vi "Events With Slow Digital Input.vi"() -> ()   [LabVIEW 2013]
uses:
  Version Token.ctl
  APU/Settings.ctl
  APU/Input.ctl
  APU/Output.ctl
  APU/Shared Settings.ctl
  ECU Event/Timing/Measure Output.ctl
  ECU Event/Timing/Measure Settings.ctl
  ECU Event/Timing/Capture Output.ctl
  <vilib>/Platform/TimedLoop/XDataNode/timing_clust.ctl
  <vilib>/Platform/TimedLoop/XDataNode/nitl_modes.ctl
  <vilib>/Platform/TimedLoop/XDataNode/wakeup.ctl
  ECU Event/Timing/Capture Settings.ctl
  <vilib>/rvi/Emulation/niFpgaSctlEmulationGetInTimedLoop.vi
  <vilib>/rvi/Emulation/niFpgaEmulationReportErrorSimple.vi
  <vilib>/rvi/Emulation/niFpgaGetClockAttributes.vi
  <vilib>/rvi/Emulation/niFpgaCriticalErrorInLSC.vi
  <vilib>/rvi/eio/common/nirviEmuTemplateMethod_errors.vi
  ECU Event/Timing/Measure Events (Non-40MHz).vi
  <vilib>/Platform/TimedLoop/XDataNode/XDataNode.xnode
  <vilib>/eio/EIONode/EIONode.xnode
  APU/APU.lvlib
  <vilib>/Platform/TimedLoop/XDataNode/XDNodeRunTimeDep.lvlib
  ECU Event/Timing/ECU Event Timing.lvlib
  Engine Simulation Toolkit.lvlib
panel:
  in  "go.apu 1":bool
  out "capture.Multi Event DIO 15.Event 4":T1
  out "capture.Multi Event DIO 15.Event 3":T1
  out "capture.Multi Event DIO 15.Event 2":T1
  out "capture.Multi Event DIO 14.Event 4":T1
  out "capture.Multi Event DIO 14.Event 3":T1
  out "capture.Multi Event DIO 14.Event 2":T1
  out "capture.Multi Event DIO 13.Event 4":T1
  out "capture.Multi Event DIO 13.Event 3":T1
  out "capture.Multi Event DIO 13.Event 2":T1
  out "capture.Multi Event DIO 12.Event 4":T1
  out "capture.Multi Event DIO 12.Event 3":T1
  out "capture.Multi Event DIO 12.Event 2":T1
  out "capture.Multi Event DIO 11.Event 4":T1
  out "capture.Multi Event DIO 11.Event 3":T1
  out "capture.Multi Event DIO 11.Event 2":T1
  out "capture.Multi Event DIO 10.Event 4":T1
  out "capture.Multi Event DIO 10.Event 3":T1
  out "capture.Multi Event DIO 10.Event 2":T1
  out "capture.Multi Event DIO 10.Event 1":T1
  out "capture.Multi Event DIO 11.Event 1":T1
  out "capture.Multi Event DIO 12.Event 1":T1
  out "capture.Multi Event DIO 13.Event 1":T1
  out "capture.Multi Event DIO 14.Event 1":T1
  out "capture.Multi Event DIO 15.Event 1":T1
  in  "settings.Multi Event DIO 10":T2
  in  "settings.Multi Event DIO 11":T2
  in  "settings.Multi Event DIO 12":T2
  in  "settings.Multi Event DIO 13":T2
  in  "settings.Multi Event DIO 14":T2
  in  "settings.Multi Event DIO 15":T2
  out "status.Multi Event DIO 10":T3
  out "status.Multi Event DIO 11":T3
  out "status.Multi Event DIO 12":T3
  out "status.Multi Event DIO 13":T3
  out "status.Multi Event DIO 14":T3
  out "status.Multi Event DIO 15":T3
  out "capture.Event DIO 4.Event 1":T1
  out "capture.Event DIO 5.Event 1":T1
  out "capture.Event DIO 6.Event 1":T1
  out "capture.Event DIO 7.Event 1":T1
  out "capture.Event DIO 8.Event 1":T1
  out "capture.Event DIO 9.Event 1":T1
  in  "settings.Event DIO 4":T2
  in  "settings.Event DIO 5":T2
  in  "settings.Event DIO 6":T2
  in  "settings.Event DIO 7":T2
  in  "settings.Event DIO 8":T2
  in  "settings.Event DIO 9":T2
  out "status.Event DIO 4":T3
  out "status.Event DIO 5":T3
  out "status.Event DIO 6":T3
  out "status.Event DIO 7":T3
  out "status.Event DIO 8":T3
  out "status.Event DIO 9":T3
  in  "shared settings.apu 1":T4 {"cycle start" format="%#.15g"}
  out "output.apu 1":T5 caption="output"
  in  "input.apu 1":T6={"desired speed"=0.0, "reset"=TRUE} caption="input"
  in  "settings.apu 1":T7 caption="settings"
  in  "est.version":T8
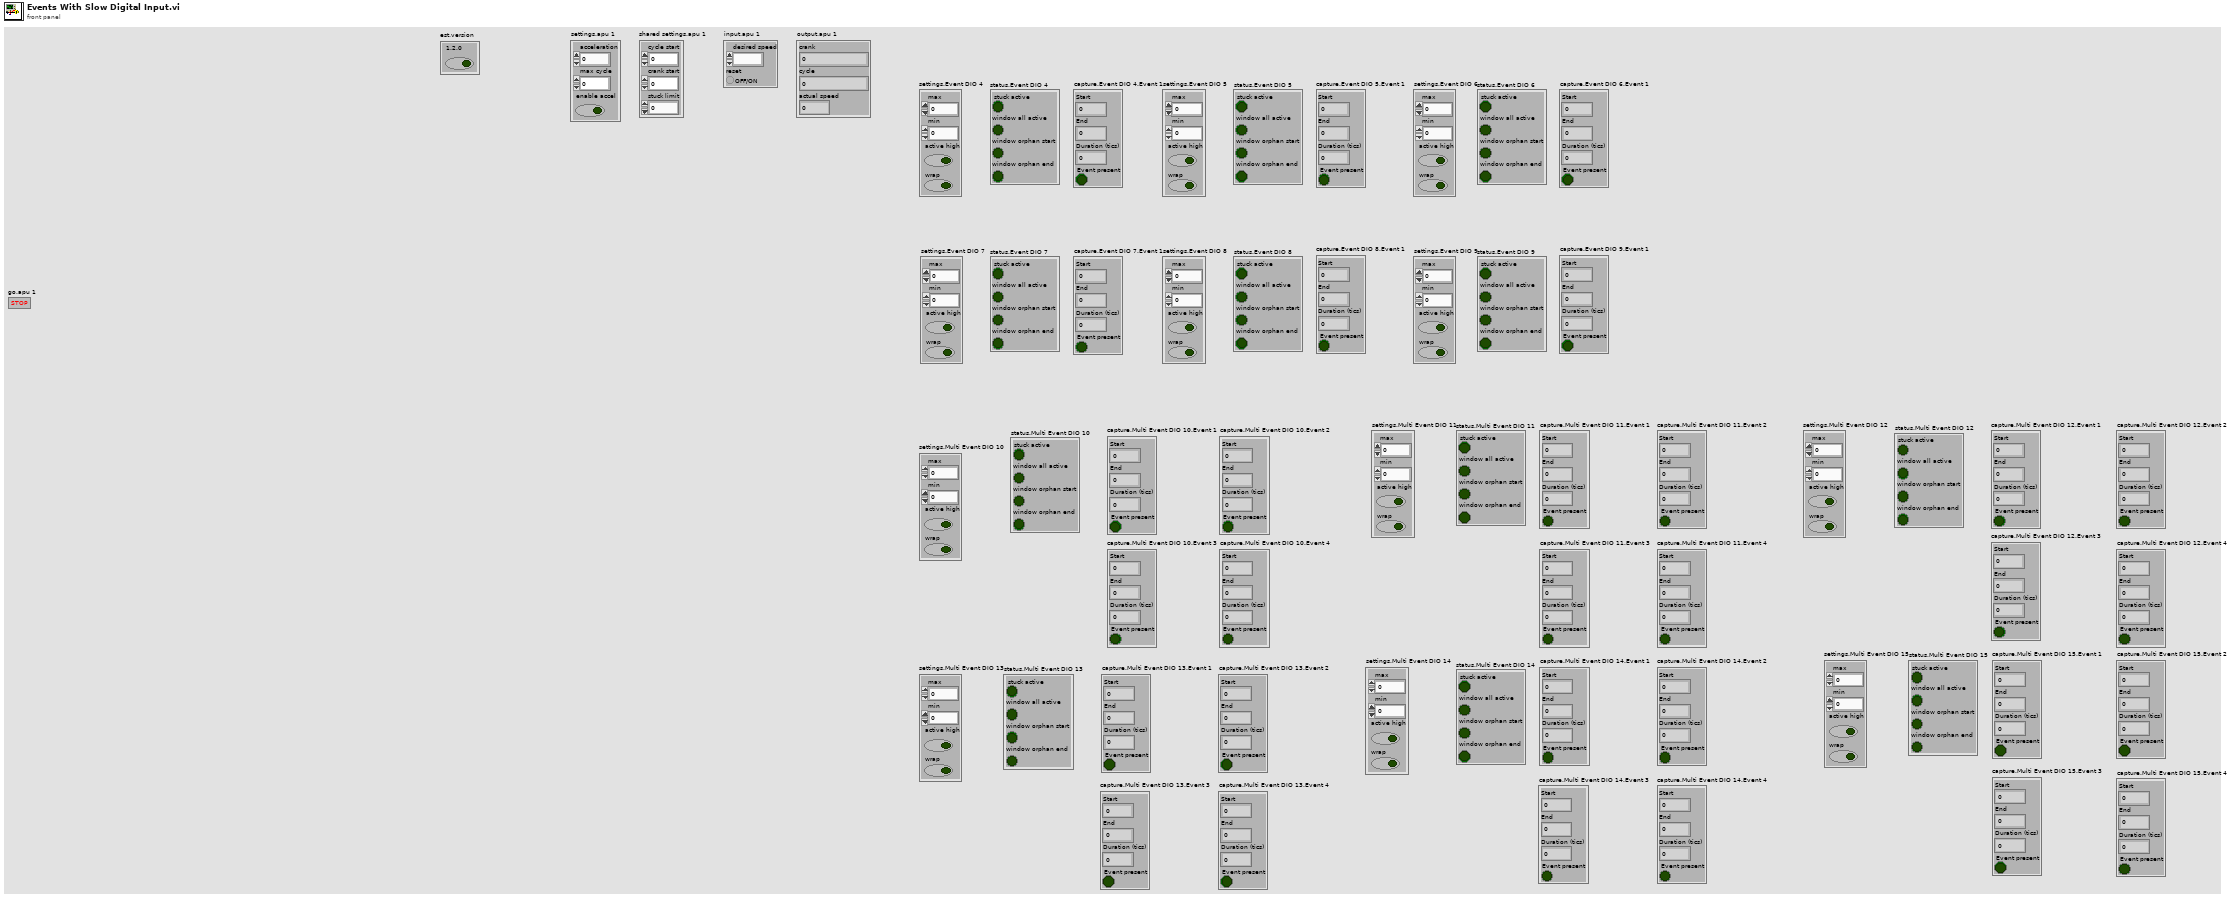
[diagram p1: front panel]
types:
  T1 = typedef "Engine Simulation Toolkit.lvlib/ECU Event Timing.lvlib/Capture Output.ctl" = cluster{"Start":u16, "End":u16, "Duration (tics)":fxp<+,18,18>, "Event present":bool}
  T2 = typedef "Engine Simulation Toolkit.lvlib/ECU Event Timing.lvlib/Measure Settings.ctl" = cluster{"max":u16, "min":u16, "active high":bool, "wrap":bool}
  T3 = typedef "Engine Simulation Toolkit.lvlib/ECU Event Timing.lvlib/Measure Output.ctl" = cluster{"stuck active":bool, "window all active":bool, "window orphan start":bool, "window orphan end":bool}
  T4 = typedef "Engine Simulation Toolkit.lvlib/APU.lvlib/Shared Settings.ctl" = cluster{"cycle start":fxp<+,2,2>, "crank start":u16, "stuck limit":fxp<+,18,18>}
  T5 = typedef "Engine Simulation Toolkit.lvlib/APU.lvlib/Output.ctl" = cluster{"crank":u16, "cycle":u16, "actual speed":fxp<+/-,23,2>}
  T6 = typedef "Engine Simulation Toolkit.lvlib/APU.lvlib/Input.ctl" = cluster{"desired speed":fxp<+/-,23,2>, "reset":bool}
  T7 = typedef "Engine Simulation Toolkit.lvlib/APU.lvlib/Settings.ctl" = cluster{"acceleration":fxp<+,18,-20>, "max cycle":fxp<+,2,2>, "enable accel":bool}
  T8 = typedef "Engine Simulation Toolkit.lvlib/Version Token.ctl" = cluster{"1.2.0":bool}
  T9 = typedef "XDNodeRunTimeDep.lvlib/timing_clust.ctl" = cluster{"Expected End [f-1]":u64, "Actual End [f-1]":u64, "Finished Late? [f-1]":bool, "Expected End [i-1]":u64, "Actual End [i-1]":u64, "Finished Late? [i-1]":bool, "Expected Start [i]":u64, "Actual Start [i]":u64, "Expected Start [f]":u64, "Actual Start [f]":u64, "Source Name":string, "Structure Name":string, "Period":i64, "Deadline":i64, "Offset":i64, "Start":i64, "Priority":i32, "Timeout":i32, "Mode":T10, "Wakeup Reason":T11, "Error":errorcluster, "Source Type":string, "Secondary Source Type":string, "Global End Time":u64, "Global Start Time":u64, "Frame Duration":u64, "Iteration Duration":u64, "Assigned CPU":i32, "I/O Scan Engine Mode":u32}
  T10 = typedef "XDNodeRunTimeDep.lvlib/nitl_modes.ctl" = enum32{"No Change", "Process missed periods, maintain original phase", "Discard missed periods, maintain original phase", "Process missed periods, ignore original phase", "Discard missed periods, ignore original phase"}
  T11 = typedef "XDNodeRunTimeDep.lvlib/wakeup.ctl" = enum32{"Normal", "Aborted", "Asynchronous wakeup", "Timing source error", "Timed loop error", "Timeout"}
  T12 = typedef "Engine Simulation Toolkit.lvlib/APU.lvlib/Register Bus.ctl" = cluster{"Speed":refnum<k21>, "Crank Angle":refnum<k21>, "Cycle Angle":refnum<k21>, "Crank Count":refnum<k21>, "Cycle Count":refnum<k21>, "1.25 MHz Counter":refnum<k21>, "shared settings":T4}
  T13 = typedef "Engine Simulation Toolkit.lvlib/ECU Event Timing.lvlib/Capture Settings.ctl" = u8
  T14 = typedef "Engine Simulation Toolkit.lvlib/ECU Event Timing.lvlib/Measured Data.ctl" = cluster{"start":u16, "end":u16, "duration (tics)":fxp<+,18,18>, "window end":bool, "window begin":bool, "pulse end":bool, "pulse #":u8}
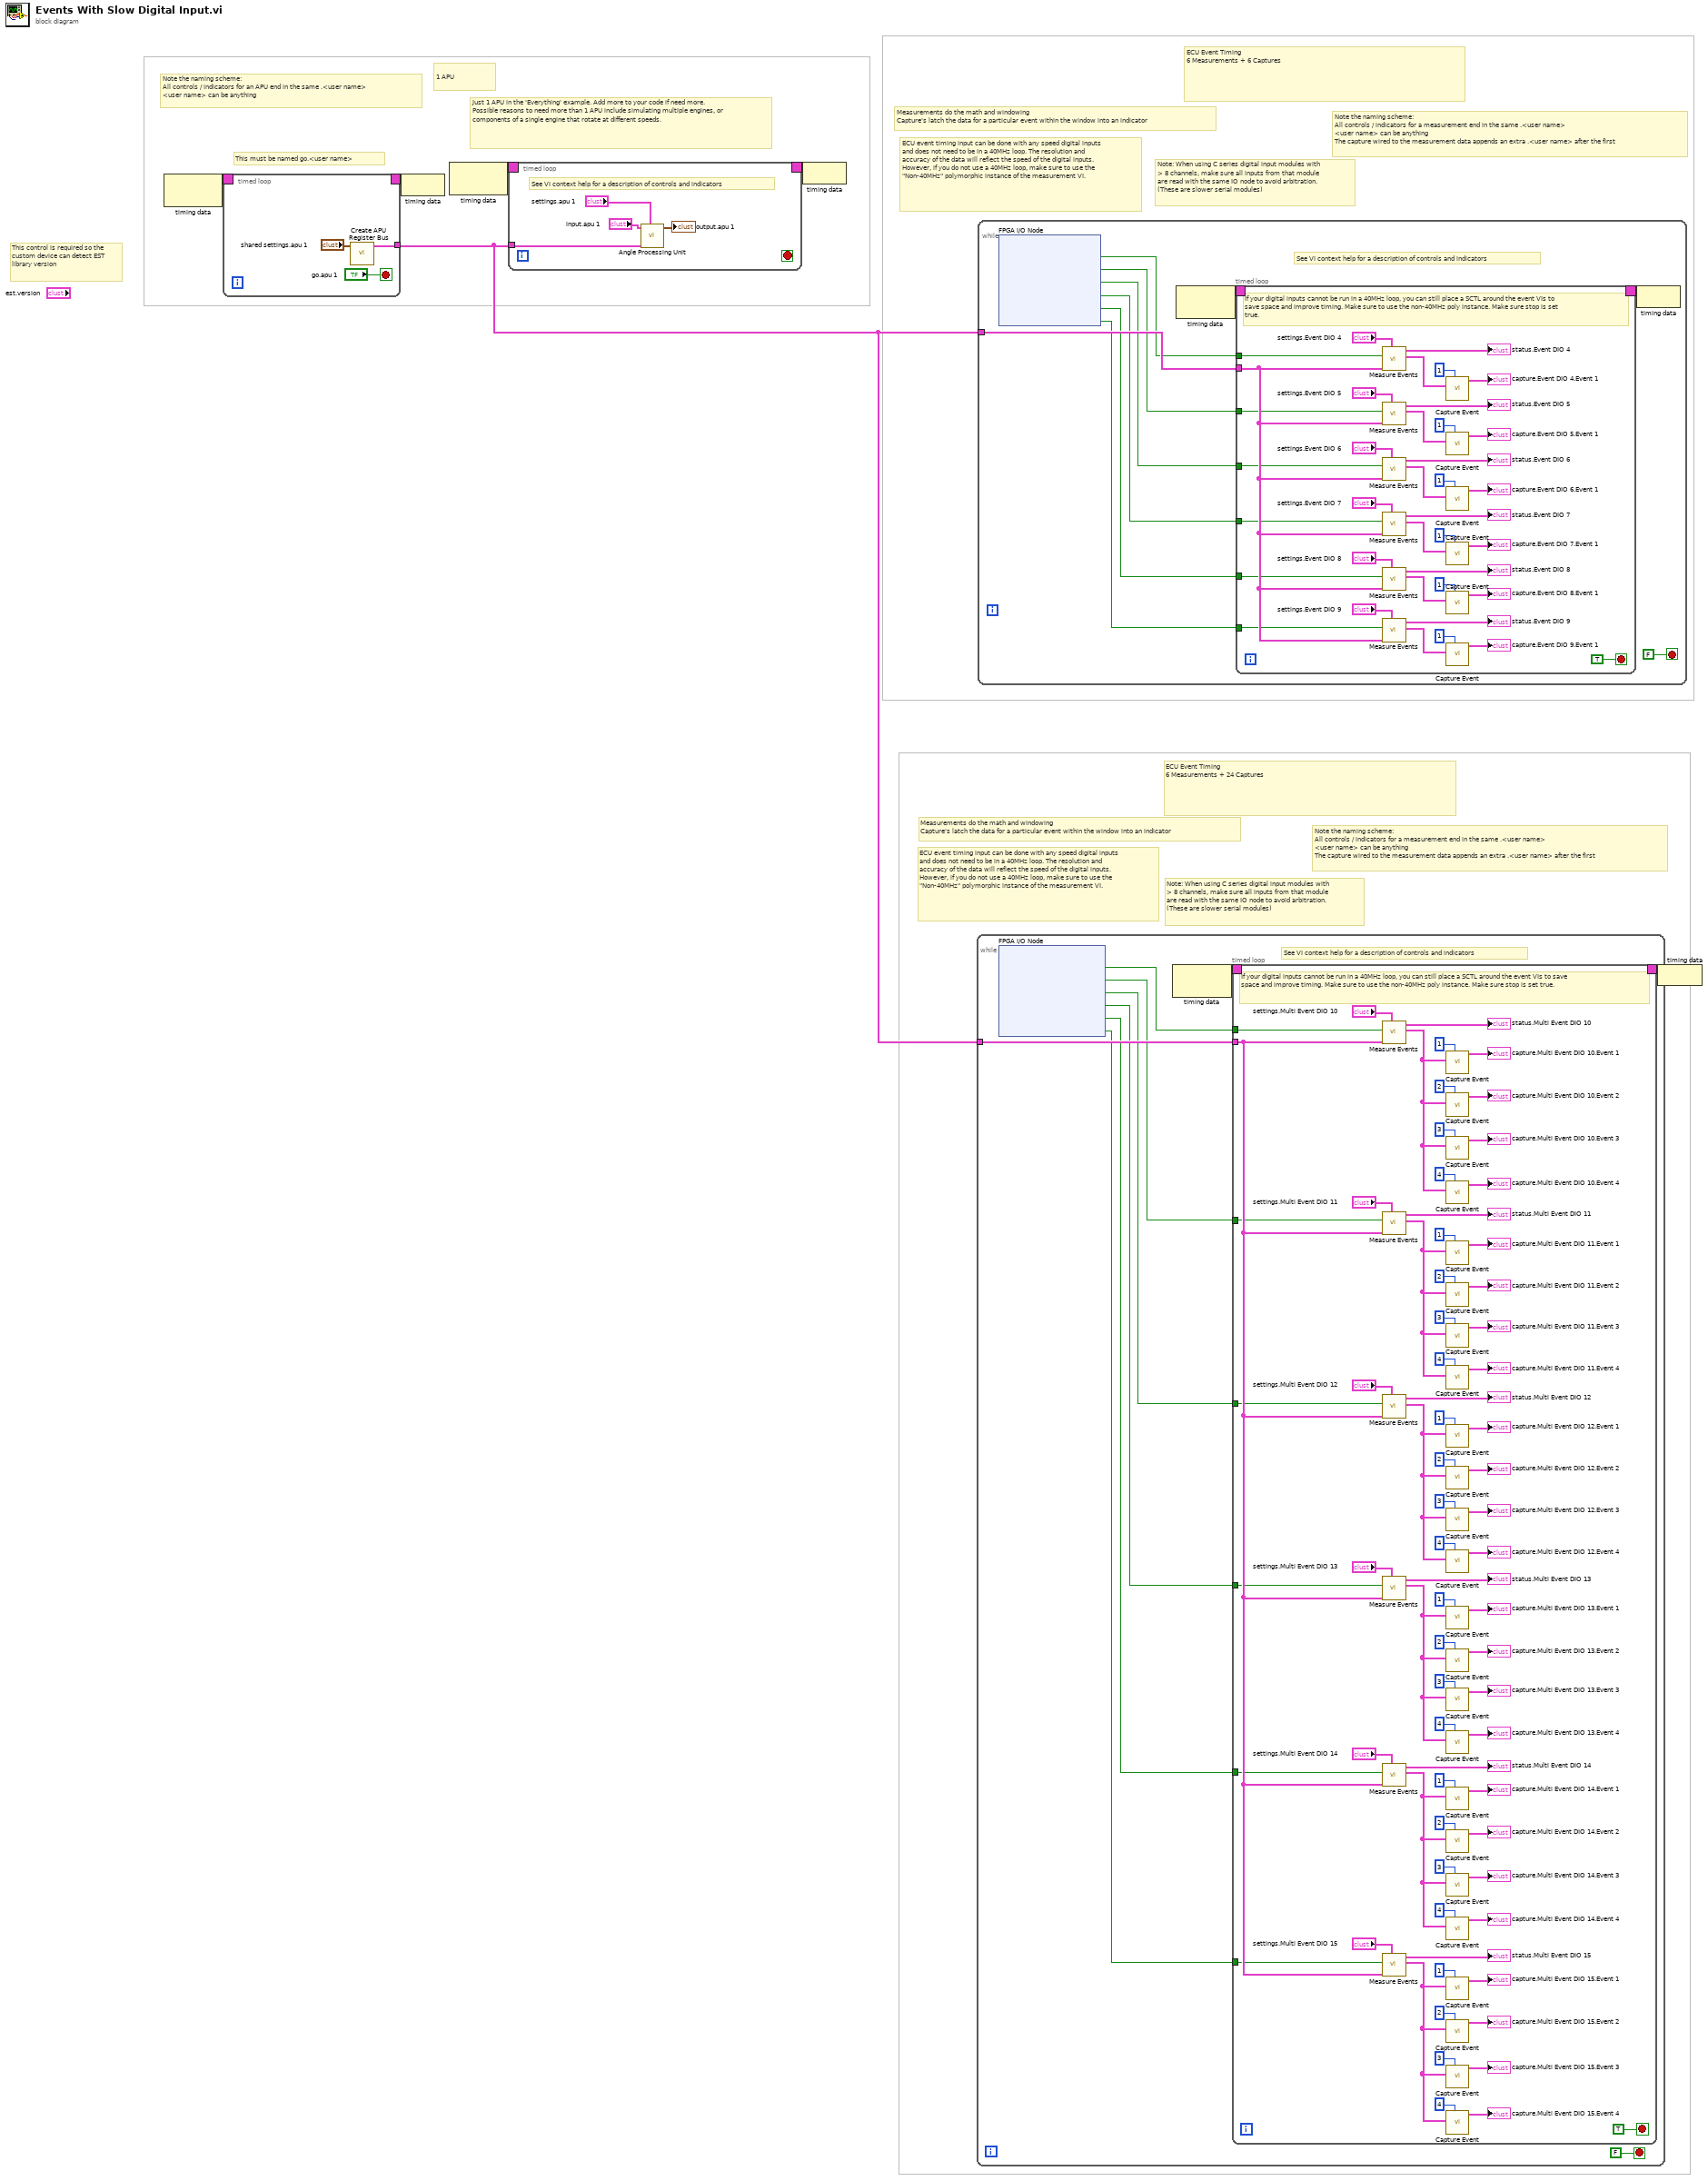
[diagram p0: block diagram]
diagram:
  # "ECU event timing input can be done with any speed digital inputs and does not need to be in a 40MHz loop. The resolution and accuracy of the data will reflect the speed of the digital inputs. However, if you do not use a 40MHz loop, make sure to use the \"Non-40MHz\" polymorphic instance of the measurement VI."
  # "This must be named go.<user name>"
  # "Note: When using C series digital input modules with > 8 channels, make sure all inputs from that module are read with the same IO node to avoid arbitration. (These are slower serial modules)"
  # "Measurements do the math and windowing\nCapture's latch the data for a particular event within the window into an indicator"
  # "ECU Event Timing\n6 Measurements + 24 Captures"
  # "Note the naming scheme: \nAll controls / indicators for a measurement end in the same .<user name>\n<user name> can be anything\nThe capture wired to the measurement data appends an extra .<user name> after the first"
  # "Note: When using C series digital input modules with > 8 channels, make sure all inputs from that module are read with the same IO node to avoid arbitration. (These are slower serial modules)"
  # "Measurements do the math and windowing\nCapture's latch the data for a particular event within the window into an indicator"
  # "ECU Event Timing\n6 Measurements + 6 Captures"
  # "Note the naming scheme: \nAll controls / indicators for a measurement end in the same .<user name>\n<user name> can be anything\nThe capture wired to the measurement data appends an extra .<user name> after the first"
  # "ECU event timing input can be done with any speed digital inputs and does not need to be in a 40MHz loop. The resolution and accuracy of the data will reflect the speed of the digital inputs. However, if you do not use a 40MHz loop, make sure to use the \"Non-40MHz\" polymorphic instance of the measurement VI."
  # "1 APU"
  # "Note the naming scheme: \nAll controls / indicators for an APU end in the same .<user name>\n<user name> can be anything"
  # "Just 1 APU in the 'Everything' example. Add more to your code if need more. Possible reasons to need more than 1 APU include simulating multiple engines, or components of a single engine that rotate at different speeds."
  # "This control is required so the custom device can detect EST library version"
  n1 = node-c288() -> (w2:T9)  [unwired: 1 in]
  n2 = timed-loop {
    timing: w2 -> [_]
    timing-out: [_] -> w1
    tunnel: [w7] -> w3
    stop <- "go.apu 1" stop-if-true
    n3 = call "Create APU Register Bus.vi"("shared settings.<user name>"="shared settings.apu 1") -> ("register bus"=w7:T12)  [unwired: 10 in]
  }
  n4 = node-c288(w1) -> ()
  n5 = node-c288() -> (w5:T9)  [unwired: 1 in]
  n6 = timed-loop {
    timing: w5 -> [_]
    timing-out: [_] -> w4
    tunnel: w3 -> [w11]
    stop <- _ stop-if-true
    # "See VI context help for a description of controls and indicators"
    n7 = call "Angle Processing Unit.vi"("settings.<user name>"="settings.apu 1", "register bus"=w11, "input.<user name>"="input.apu 1") -> ("output.<user name>"=→"output.apu 1":T5)  [unwired: 8 in]
  }
  n8 = node-c288(w4) -> ()
  n9 = while {
    tunnel: w3 -> [w26]
    stop <- FALSE stop-if-true
    # "See VI context help for a description of controls and indicators"
    n10 = xnode "FPGA I/O Node"() -> ("Connector0/DIO10"=w25:bool, "Connector0/DIO11"=w24:bool, "Connector0/DIO12"=w23:bool, "Connector0/DIO13"=w22:bool, "Connector0/DIO14"=w21:bool, "Connector0/DIO15"=w20:bool)  [unwired: 6 in, 6 out]
    n11 = node-c288() -> (w18:T9)  [unwired: 1 in]
    n12 = timed-loop {
      timing: w18 -> [_]
      timing-out: [_] -> w17
      tunnel: w26 -> [w94]
      tunnel: w25 -> [w81]
      tunnel: w24 -> [w80]
      tunnel: w23 -> [w79]
      tunnel: w22 -> [w78]
      tunnel: w21 -> [w77]
      tunnel: w20 -> [w76]
      stop <- TRUE stop-if-true
      # "If your digital inputs cannot be run in a 40MHz loop, you can still place a SCTL around the event VIs to save space and improve timing. Make sure to use the non-40MHz poly instance. Make sure stop is set true."
      n13 = call-poly "Measure Events.vi"("settings.<user name>"="settings.Multi Event DIO 10", "register bus"=w94, "event"=w81) -> ("measured data"=w63:T14, "status.<user name>"=→"status.Multi Event DIO 10":T3)  [unwired: 7 in]
      n14 = call-poly "Measure Events.vi"("settings.<user name>"="settings.Multi Event DIO 11", "register bus"=w94, "event"=w80) -> ("measured data"=w56:T14, "status.<user name>"=→"status.Multi Event DIO 11":T3)  [unwired: 7 in]
      n15 = call-poly "Measure Events.vi"("settings.<user name>"="settings.Multi Event DIO 12", "register bus"=w94, "event"=w79) -> ("measured data"=w49:T14, "status.<user name>"=→"status.Multi Event DIO 12":T3)  [unwired: 7 in]
      n16 = call-poly "Measure Events.vi"("settings.<user name>"="settings.Multi Event DIO 13", "register bus"=w94, "event"=w78) -> ("measured data"=w42:T14, "status.<user name>"=→"status.Multi Event DIO 13":T3)  [unwired: 7 in]
      n17 = call-poly "Measure Events.vi"("settings.<user name>"="settings.Multi Event DIO 14", "register bus"=w94, "event"=w77) -> ("measured data"=w35:T14, "status.<user name>"=→"status.Multi Event DIO 14":T3)  [unwired: 7 in]
      n18 = call-poly "Measure Events.vi"("settings.<user name>"="settings.Multi Event DIO 15", "register bus"=w94, "event"=w76) -> ("measured data"=w28:T14, "status.<user name>"=→"status.Multi Event DIO 15":T3)  [unwired: 7 in]
      n19 = call "Capture Event.vi"("event # to capture"=T13 1 ("Settings.spark 1 shot 1"), "measured data"=w63) -> ("capture.<user name>"=→"capture.Multi Event DIO 10.Event 1":T1)  [unwired: 9 in]
      n20 = call "Capture Event.vi"("event # to capture"=T13 2 ("Settings.spark 1 shot 1"), "measured data"=w63) -> ("capture.<user name>"=→"capture.Multi Event DIO 10.Event 2":T1)  [unwired: 9 in]
      n21 = call "Capture Event.vi"("event # to capture"=T13 3 ("Settings.spark 1 shot 1"), "measured data"=w63) -> ("capture.<user name>"=→"capture.Multi Event DIO 10.Event 3":T1)  [unwired: 9 in]
      n22 = call "Capture Event.vi"("event # to capture"=T13 4 ("Settings.spark 1 shot 1"), "measured data"=w63) -> ("capture.<user name>"=→"capture.Multi Event DIO 10.Event 4":T1)  [unwired: 9 in]
      n23 = call "Capture Event.vi"("event # to capture"=T13 1 ("Settings.spark 2 shot 1"), "measured data"=w56) -> ("capture.<user name>"=→"capture.Multi Event DIO 11.Event 1":T1)  [unwired: 9 in]
      n24 = call "Capture Event.vi"("event # to capture"=T13 2 ("Settings.spark 2 shot 1"), "measured data"=w56) -> ("capture.<user name>"=→"capture.Multi Event DIO 11.Event 2":T1)  [unwired: 9 in]
      n25 = call "Capture Event.vi"("event # to capture"=T13 3 ("Settings.spark 2 shot 1"), "measured data"=w56) -> ("capture.<user name>"=→"capture.Multi Event DIO 11.Event 3":T1)  [unwired: 9 in]
      n26 = call "Capture Event.vi"("event # to capture"=T13 4 ("Settings.spark 2 shot 1"), "measured data"=w56) -> ("capture.<user name>"=→"capture.Multi Event DIO 11.Event 4":T1)  [unwired: 9 in]
      n27 = call "Capture Event.vi"("event # to capture"=T13 1 ("Settings.spark 3 shot 1"), "measured data"=w49) -> ("capture.<user name>"=→"capture.Multi Event DIO 12.Event 1":T1)  [unwired: 9 in]
      n28 = call "Capture Event.vi"("event # to capture"=T13 2 ("Settings.spark 3 shot 1"), "measured data"=w49) -> ("capture.<user name>"=→"capture.Multi Event DIO 12.Event 2":T1)  [unwired: 9 in]
      n29 = call "Capture Event.vi"("event # to capture"=T13 3 ("Settings.spark 3 shot 1"), "measured data"=w49) -> ("capture.<user name>"=→"capture.Multi Event DIO 12.Event 3":T1)  [unwired: 9 in]
      n30 = call "Capture Event.vi"("event # to capture"=T13 4 ("Settings.spark 3 shot 1"), "measured data"=w49) -> ("capture.<user name>"=→"capture.Multi Event DIO 12.Event 4":T1)  [unwired: 9 in]
      n31 = call "Capture Event.vi"("event # to capture"=T13 1 ("Settings.spark 4 shot 1"), "measured data"=w42) -> ("capture.<user name>"=→"capture.Multi Event DIO 13.Event 1":T1)  [unwired: 9 in]
      n32 = call "Capture Event.vi"("event # to capture"=T13 2 ("Settings.spark 4 shot 1"), "measured data"=w42) -> ("capture.<user name>"=→"capture.Multi Event DIO 13.Event 2":T1)  [unwired: 9 in]
      n33 = call "Capture Event.vi"("event # to capture"=T13 3 ("Settings.spark 4 shot 1"), "measured data"=w42) -> ("capture.<user name>"=→"capture.Multi Event DIO 13.Event 3":T1)  [unwired: 9 in]
      n34 = call "Capture Event.vi"("event # to capture"=T13 4 ("Settings.spark 4 shot 1"), "measured data"=w42) -> ("capture.<user name>"=→"capture.Multi Event DIO 13.Event 4":T1)  [unwired: 9 in]
      n35 = call "Capture Event.vi"("event # to capture"=T13 1 ("Settings.spark 5 shot 1"), "measured data"=w35) -> ("capture.<user name>"=→"capture.Multi Event DIO 14.Event 1":T1)  [unwired: 9 in]
      n36 = call "Capture Event.vi"("event # to capture"=T13 2 ("Settings.spark 5 shot 1"), "measured data"=w35) -> ("capture.<user name>"=→"capture.Multi Event DIO 14.Event 2":T1)  [unwired: 9 in]
      n37 = call "Capture Event.vi"("event # to capture"=T13 3 ("Settings.spark 5 shot 1"), "measured data"=w35) -> ("capture.<user name>"=→"capture.Multi Event DIO 14.Event 3":T1)  [unwired: 9 in]
      n38 = call "Capture Event.vi"("event # to capture"=T13 4 ("Settings.spark 5 shot 1"), "measured data"=w35) -> ("capture.<user name>"=→"capture.Multi Event DIO 14.Event 4":T1)  [unwired: 9 in]
      n39 = call "Capture Event.vi"("event # to capture"=T13 1 ("Settings.spark 6 shot 1"), "measured data"=w28) -> ("capture.<user name>"=→"capture.Multi Event DIO 15.Event 1":T1)  [unwired: 9 in]
      n40 = call "Capture Event.vi"("event # to capture"=T13 2 ("Settings.spark 6 shot 1"), "measured data"=w28) -> ("capture.<user name>"=→"capture.Multi Event DIO 15.Event 2":T1)  [unwired: 9 in]
      n41 = call "Capture Event.vi"("event # to capture"=T13 3 ("Settings.spark 6 shot 1"), "measured data"=w28) -> ("capture.<user name>"=→"capture.Multi Event DIO 15.Event 3":T1)  [unwired: 9 in]
      n42 = call "Capture Event.vi"("event # to capture"=T13 4 ("Settings.spark 6 shot 1"), "measured data"=w28) -> ("capture.<user name>"=→"capture.Multi Event DIO 15.Event 4":T1)  [unwired: 9 in]
    }
    n43 = node-c288(w17) -> ()
  }
  n44 = while {
    tunnel: w3 -> [w114]
    stop <- FALSE stop-if-true
    # "See VI context help for a description of controls and indicators"
    n45 = xnode "FPGA I/O Node"() -> ("Connector0/DIO4"=w113:bool, "Connector0/DIO5"=w112:bool, "Connector0/DIO6"=w111:bool, "Connector0/DIO7"=w110:bool, "Connector0/DIO8"=w109:bool, "Connector0/DIO9"=w108:bool)  [unwired: 6 in, 6 out]
    n46 = node-c288() -> (w106:T9)  [unwired: 1 in]
    n47 = timed-loop {
      timing: w106 -> [_]
      timing-out: [_] -> w105
      tunnel: w114 -> [w146]
      tunnel: w113 -> [w127]
      tunnel: w112 -> [w126]
      tunnel: w111 -> [w125]
      tunnel: w110 -> [w124]
      tunnel: w109 -> [w123]
      tunnel: w108 -> [w122]
      stop <- TRUE stop-if-true
      # "If your digital inputs cannot be run in a 40MHz loop, you can still place a SCTL around the event VIs to save space and improve timing. Make sure to use the non-40MHz poly instance. Make sure stop is set true."
      n48 = call-poly "Measure Events.vi"("settings.<user name>"="settings.Event DIO 4", "register bus"=w146, "event"=w127) -> ("measured data"=w145:T14, "status.<user name>"=→"status.Event DIO 4":T3)  [unwired: 7 in]
      n49 = call-poly "Measure Events.vi"("settings.<user name>"="settings.Event DIO 5", "register bus"=w146, "event"=w126) -> ("measured data"=w138:T14, "status.<user name>"=→"status.Event DIO 5":T3)  [unwired: 7 in]
      n50 = call-poly "Measure Events.vi"("settings.<user name>"="settings.Event DIO 6", "register bus"=w146, "event"=w125) -> ("measured data"=w137:T14, "status.<user name>"=→"status.Event DIO 6":T3)  [unwired: 7 in]
      n51 = call-poly "Measure Events.vi"("settings.<user name>"="settings.Event DIO 7", "register bus"=w146, "event"=w124) -> ("measured data"=w136:T14, "status.<user name>"=→"status.Event DIO 7":T3)  [unwired: 7 in]
      n52 = call-poly "Measure Events.vi"("settings.<user name>"="settings.Event DIO 8", "register bus"=w146, "event"=w123) -> ("measured data"=w135:T14, "status.<user name>"=→"status.Event DIO 8":T3)  [unwired: 7 in]
      n53 = call-poly "Measure Events.vi"("settings.<user name>"="settings.Event DIO 9", "register bus"=w146, "event"=w122) -> ("measured data"=w134:T14, "status.<user name>"=→"status.Event DIO 9":T3)  [unwired: 7 in]
      n54 = call "Capture Event.vi"("event # to capture"=T13 1 ("Settings.spark 1 shot 1"), "measured data"=w145) -> ("capture.<user name>"=→"capture.Event DIO 4.Event 1":T1)  [unwired: 9 in]
      n55 = call "Capture Event.vi"("event # to capture"=T13 1 ("Settings.spark 2 shot 1"), "measured data"=w138) -> ("capture.<user name>"=→"capture.Event DIO 5.Event 1":T1)  [unwired: 9 in]
      n56 = call "Capture Event.vi"("event # to capture"=T13 1 ("Settings.spark 3 shot 1"), "measured data"=w137) -> ("capture.<user name>"=→"capture.Event DIO 6.Event 1":T1)  [unwired: 9 in]
      n57 = call "Capture Event.vi"("event # to capture"=T13 1 ("Settings.spark 4 shot 1"), "measured data"=w136) -> ("capture.<user name>"=→"capture.Event DIO 7.Event 1":T1)  [unwired: 9 in]
      n58 = call "Capture Event.vi"("event # to capture"=T13 1 ("Settings.spark 5 shot 1"), "measured data"=w135) -> ("capture.<user name>"=→"capture.Event DIO 8.Event 1":T1)  [unwired: 9 in]
      n59 = call "Capture Event.vi"("event # to capture"=T13 1 ("Settings.spark 6 shot 1"), "measured data"=w134) -> ("capture.<user name>"=→"capture.Event DIO 9.Event 1":T1)  [unwired: 9 in]
    }
    n60 = node-c288(w105) -> ()
  }
